vi "Target Data Global.vi"() -> ()   [LabVIEW 2014]
uses:
  Target Specific Data.ctl
panel:
  in  "VeriStand Already Startup EXE at %s":string="VeriStand Already Startup EXE at %s"
  in  "Skipping Target at %s":string="Skipping Target at %s"
  in  "Done!":string="Done!"
  in  "Restarting Target":string="Restarting Target..."
  in  "Sending INI/Conf File":string="Sending INI/Conf File..."
  in  "Modifying Tokens":string="Modifying Tokens..."
  in  "Retrieving INI/Conf File":string="Retrieving INI/Conf File..."
  in  "Verifying NI VeriStand is Installed":string="Verifying NI VeriStand is Installed..."
  in  "Opening WebDAV Connection":string="Opening WebDAV Connection..."
  in  "Reading System Definition":string="Reading System Definition..."
  in  "Linux Specific Data":T1={"VS EXE Dir Uri"="/home/lvuser/natinst/bin/", "ini or conf uri"="/etc/natinst/share/lvrt.conf", "ini or conf name"="lvrt.conf", "VS EXE Path"="/c/ni-rt/startup/NI VeriStand.rtexe"}
  in  "PharLap Specific Data":T1={"VS EXE Dir Uri"="/ni-rt/startup", "ini or conf uri"="ni-rt.ini", "ini or conf name"="ni-rt.ini", "VS EXE Path"="c:\\ni-rt\\startup\\NI VeriStand.rtexe"}
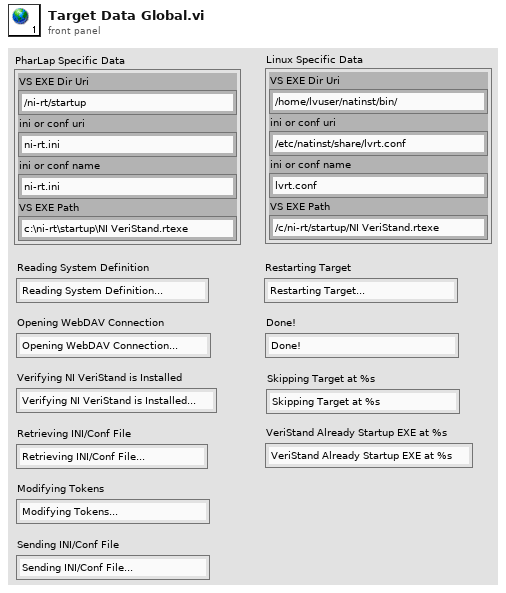
[diagram p1: front panel]
types:
  T1 = typedef "Target Specific Data.ctl" = cluster{"VS EXE Dir Uri":string, "ini or conf uri":string, "ini or conf name":string, "VS EXE Path":string}
diagram:
